vi "Merge corners.vi"(4 "New Corners":cluster{"Col":dbl, "Row":dbl}[](array[cluster]), 5 "Old corners":cluster{"Col":dbl, "Row":dbl}[](array[cluster]), 6 "Corners Matrix":T1) -> (1 "Updated Corners":cluster{"Col":dbl, "Row":dbl}[](array[cluster]), 2 "Updated Corners Matrix":T1)   [LabVIEW 2009]
uses:
  <vilib>/Analysis/Matrix/Datatypes/RealMatrix.ctl
  <vilib>/Analysis/Matrix/NI_Matrix.lvlib
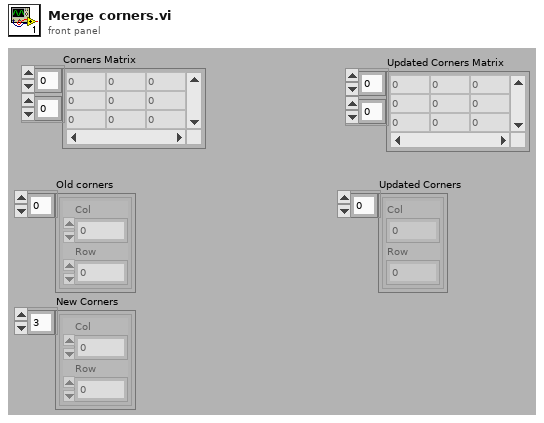
[diagram p1: front panel]
types:
  T1 = typedef "NI_Matrix.lvlib/RealMatrix.ctl" = dbl[][]
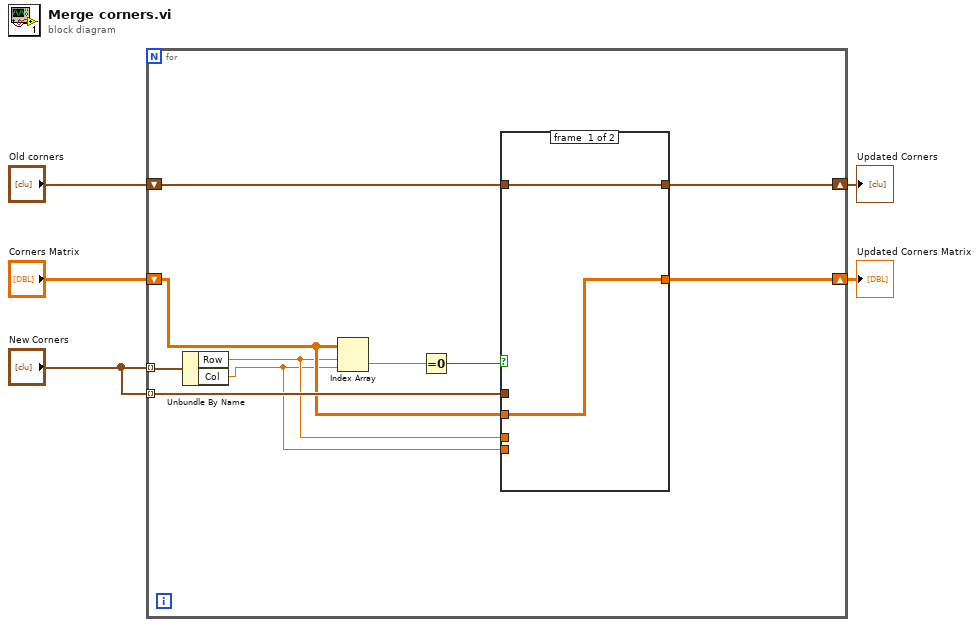
[diagram p0: block diagram]
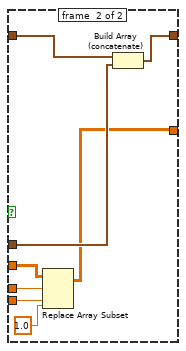
[diagram p2: hidden frame]
diagram:
  n1 = for {
    shift-right: [w11] -> w4
    shift-left: "Old corners" -> [w12]
    tunnel: "New Corners" -> [w15] mode=indexing
    tunnel: "New Corners" -> [w10] mode=indexing
    shift-right: [w9] -> w1
    shift-left: "Corners Matrix" -> [w8]
    n2 = Unbundle By Name(w15) -> ("Row"=w7:dbl, "Col"=w6:dbl)
    n3 = Index Array(array=w8, index (row)=w7, index (col)=w6) -> (element=w14:dbl)
    n4 = Equal To 0?(x=w14) -> (x = 0?=w13:bool)
    n5 = case shown="True" w13 {
      tunnel: w12 -> [w17 w25]
      tunnel: [w17 w24] -> w11
      tunnel: w10 -> [_ w23]
      tunnel: [w16 w22] -> w9
      tunnel: w8 -> [w16 w21]
      tunnel: w7 -> [_ w19]
      tunnel: w6 -> [_ w18]
      frame #0 {
      }
      frame #1 {
        n6 = Replace Array Subset(array=w21, new element=1.0 ("new element/submatrix"), index (row)=w19, index (col)=w18) -> (w22:T1)
        n7 = Build Array (concatenate)(w25, w23) -> (w24:cluster{"Col":dbl, "Row":dbl}[])
      }
    }
  }
  "Updated Corners" <- w4
  "Updated Corners Matrix" <- w1
